vi "Read file.vi"(8 "error in (no error)":errorcluster, 9 "Channel ID":u16, 10 "file path (use dialog)":path, 11 "File interpreter in":refnum<class "File interpreter.lvclass">) -> (0 "error out":errorcluster, 3 "File interpreter out":refnum<class "File interpreter.lvclass">)   [LabVIEW 2018, in "File interpreter.lvclass"]
uses:
  File interpreter.lvclass
  File interpreter.lvclass/File interpreter.ctl
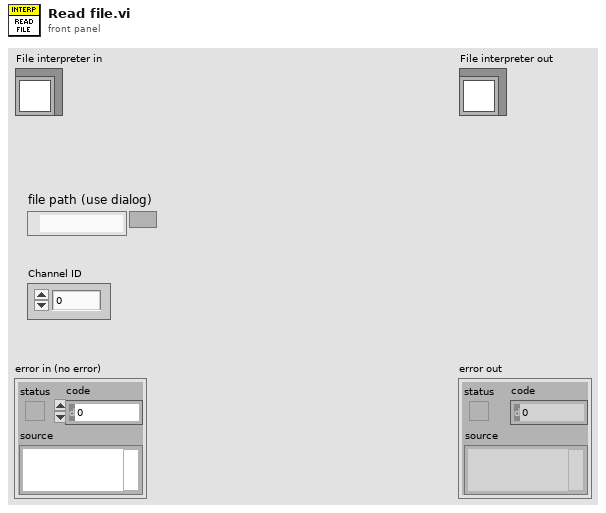
[diagram p1: front panel]
types:
  T1 = enum16{"open", "replace", "create", "open or create", "replace or create", "replace or create with confirmation"}
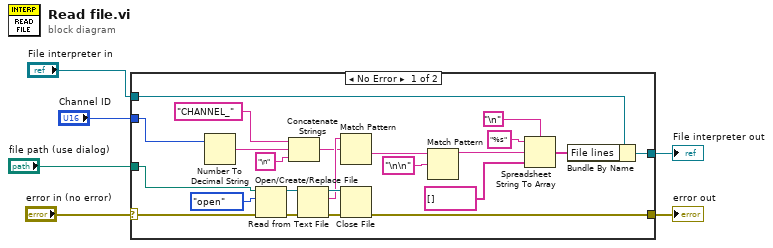
[diagram p0: block diagram]
diagram:
  n1 = case shown="No Error" "error in (no error)" {
    selector: "error in (no error)" -> [w29 w31]
    tunnel: [w20 w31] -> w5
    tunnel: [w23 w30] -> w3
    tunnel: "File interpreter in" -> [w24 w30]
    tunnel: "file path (use dialog)" -> [w28 _]
    tunnel: "Channel ID" -> [w14 _]
    frame No Error {
      n2 = Number To Decimal String(number=w14) -> (decimal integer string=w12:string)  [unwired: 1 in]
      n3 = Open/Create/Replace File(file path (use dialog)=w28, error in=w29, operation (0:open)=T1."open") -> (refnum out=w25:refnum<file>, error out=w26:errorcluster)  [unwired: 3 in, 1 out]
      n4 = Concatenate Strings("CHANNEL_", w12, "\n") -> (w10:string)
      n5 = Read from Text File(file (use dialog)=w25, error in=w26) -> (refnum out=w21:refnum<file>, text=w15:string, error out=w22:errorcluster)  [unwired: 2 in, 1 out]
      n6 = Match Pattern(string=w15, regular expression=w10) -> (after substring=w9:string)  [unwired: 1 in, 3 out]
      n7 = Close File(refnum=w21, error in=w22) -> (error out=w20:errorcluster)  [unwired: 1 out]
      n8 = Match Pattern(string=w9, regular expression="\n\n") -> (before substring=w7:string)  [unwired: 1 in, 3 out]
      n9 = Spreadsheet String To Array(delimiter (Tab)="\n", format string="%s", spreadsheet string=w7, array type (2D Dbl)=string[] []) -> (array=w16:string[])
      n10 = Bundle By Name(cluster=w24, "File lines"=w16) -> (w23:refnum<class "File interpreter.lvclass">)
    }
    frame Error {
    }
  }
  "error out" <- w5
  "File interpreter out" <- w3
